vi "enable_disable.vi"(8 "error in (no error)":errorcluster, 9 "state":T3(ring), 10 "controls":T2[](array[typedef]), 11 "control references in":T1) -> (0 "error out":errorcluster, 3 "control references out":T1)   [LabVIEW 2010]
uses:
  type_definitions/enumerations/main_control_types.ctl
  type_definitions/clusters/controls_refs.ctl
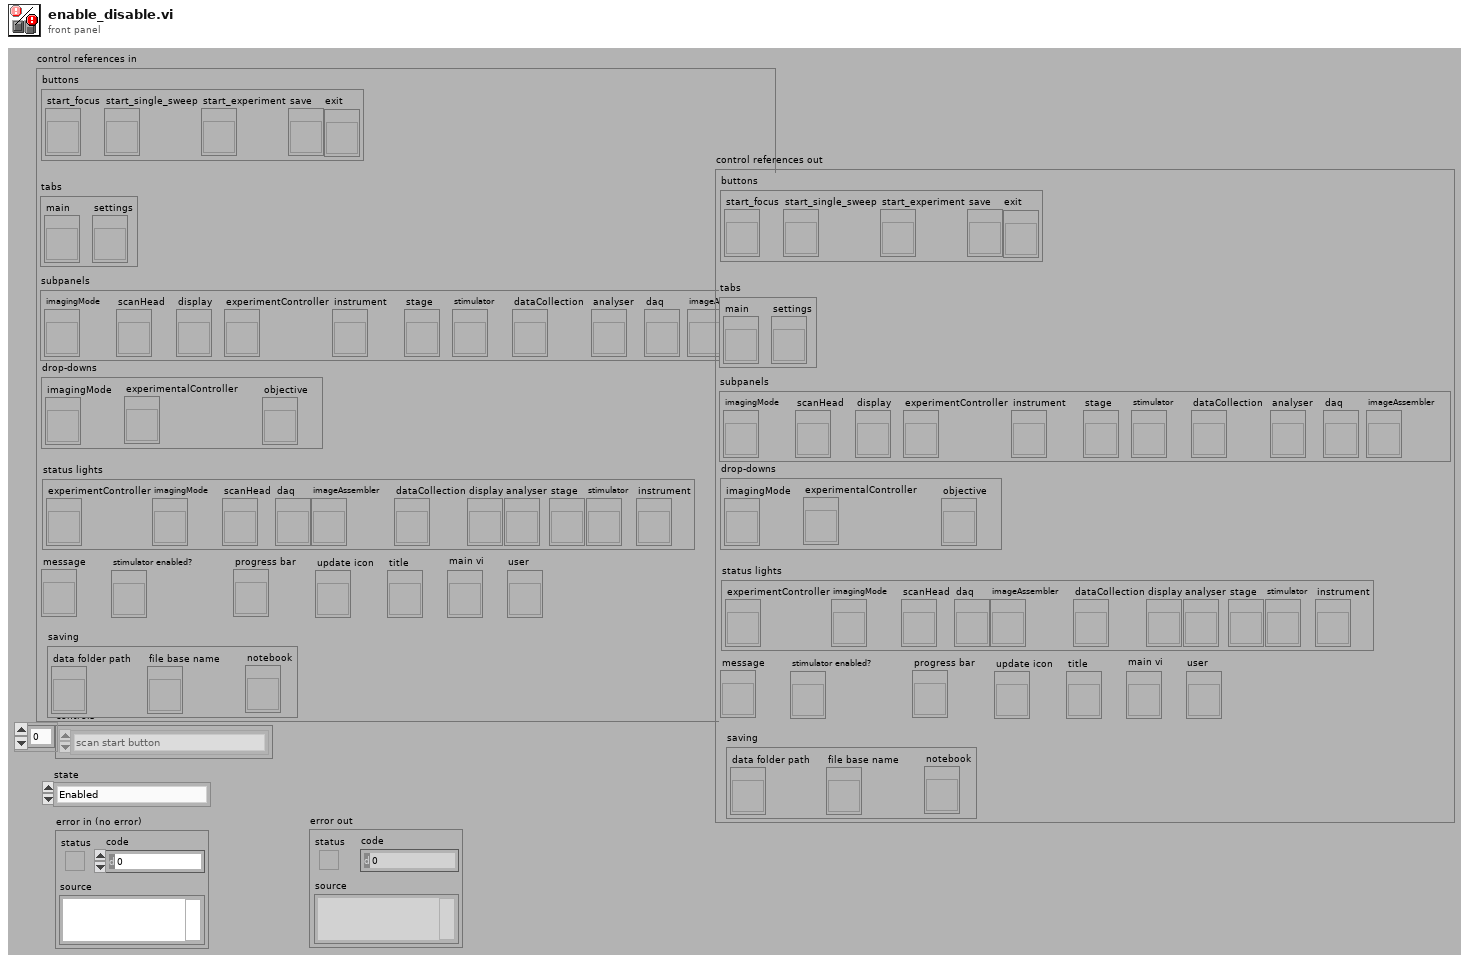
[diagram p1: front panel]
types:
  T1 = typedef "controls_refs.ctl" = cluster{"buttons":cluster{"start_focus":refnum<vi>, "start_single_sweep":refnum<vi>, "start_experiment":refnum<vi>, "save":refnum<vi>, "exit":refnum<vi>}, "tabs":cluster{"main":refnum<vi>, "settings":refnum<vi>}, "subpanels":cluster{"imagingMode":refnum<vi>, "scanHead":refnum<vi>, "display":refnum<vi>, "experimentController":refnum<vi>, "instrument":refnum<vi>, "stage":refnum<vi>, "stimulator":refnum<vi>, "dataCollection":refnum<vi>, "analyser":refnum<vi>, "daq":refnum<vi>, "imageAssembler":refnum<vi>}, "drop-downs":cluster{"imagingMode":refnum<vi>, "experimentalController":refnum<vi>, "objective":refnum<vi>}, "status lights":cluster{"experimentController":refnum<vi>, "imagingMode":refnum<vi>, "scanHead":refnum<vi>, "daq":refnum<vi>, "imageAssembler":refnum<vi>, "dataCollection":refnum<vi>, "display":refnum<vi>, "analyser":refnum<vi>, "stage":refnum<vi>, "stimulator":refnum<vi>, "instrument":refnum<vi>}, "message":refnum<vi>, "stimulator enabled?":refnum<vi>, "saving":cluster{"data folder path":refnum<vi>, "file base name":refnum<vi>, "notebook":refnum<vi>}, "progress bar":refnum<vi>, "update icon":refnum<vi>, "title":refnum<vi>, "main vi":refnum<vi>, "user":refnum<vi>}
  T2 = typedef "main_control_types.ctl" = enum16{"scan start button", "experimentController subpanel", "imagingMode subpanel", "scanHead subpanel", "dataCollection subpanel", "display subpanel", "analyser subpanel", "stimulator subpanel", "imagingMode drop-down", "experimentController drop-down", "objective drop-down", "exit button"}
  T3 = enum8{"Enabled", "Disabled", "Disabled and Grayed Out"}
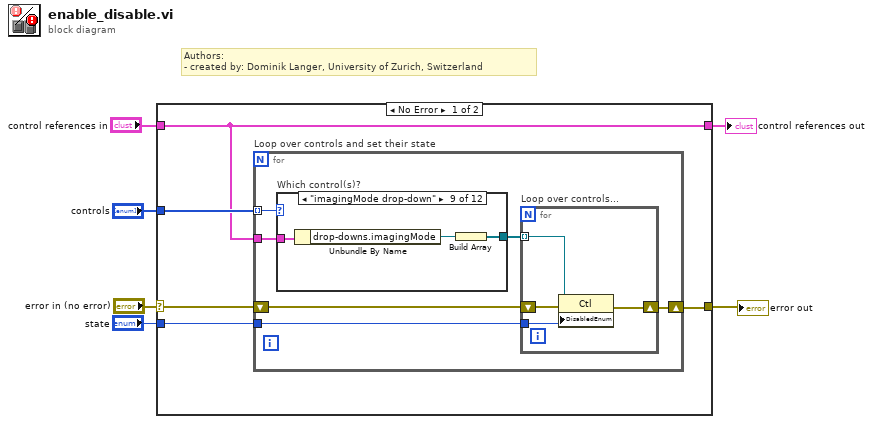
[diagram p0: block diagram]
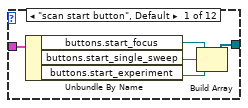
[diagram p2: hidden frame]
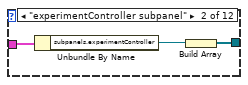
[diagram p3: hidden frame]
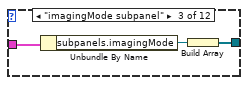
[diagram p4: hidden frame]
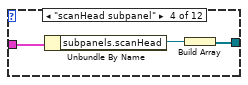
[diagram p5: hidden frame]
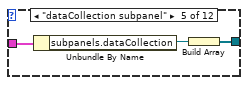
[diagram p6: hidden frame]
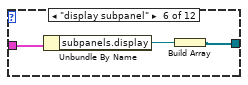
[diagram p7: hidden frame]
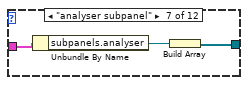
[diagram p8: hidden frame]
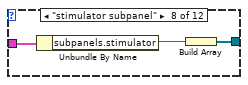
[diagram p9: hidden frame]
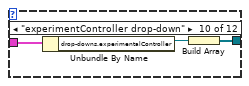
[diagram p10: hidden frame]
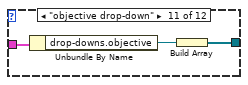
[diagram p11: hidden frame]
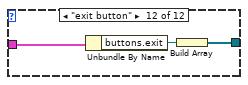
[diagram p12: hidden frame]
diagram:
  # "Authors: \n- created by: Dominik Langer, University of Zurich, Switzerland"
  n1 = case shown="No Error" "error in (no error)" {
    selector: "error in (no error)" -> [w8 w61]
    tunnel: [w10 w61] -> w5
    tunnel: "state" -> [w11 _]
    tunnel: "controls" -> [w9 _]
    tunnel: "control references in" -> [w7 w60]
    tunnel: [w7 w60] -> w1
    frame No Error {
      n2 = for "Loop over controls and set their state" {
        tunnel: w7 -> [w17]
        tunnel: w11 -> [w14]
        tunnel: w9 -> [w12] mode=indexing
        shift-right: [w13] -> w10
        shift-left: w8 -> [w16]
        n3 = case "Which control(s)?" shown="\"imagingMode drop-down\"" w12 {
          tunnel: w17 -> [w26 w29 w32 w35 w38 w41 w44 w47 w50 w53 w56 w59]
          tunnel: [w22 w27 w30 w34 w37 w39 w42 w45 w48 w52 w54 w57] -> w15
          frame "scan start button", Default {
            n4 = Unbundle By Name(w26) -> ("buttons.start_focus"=w24:refnum<vi>, "buttons.start_single_sweep"=w23:refnum<vi>, "buttons.start_experiment"=w25:refnum<vi>)
            n5 = Build Array(w24, w23, w25) -> (w22:refnum<vi>[])
          }
          frame "experimentController subpanel" {
            n6 = Unbundle By Name(w29) -> ("subpanels.experimentController"=w28:refnum<vi>)
            n7 = Build Array(w28) -> (w27:refnum<vi>[])
          }
          frame "imagingMode subpanel" {
            n8 = Unbundle By Name(w32) -> ("subpanels.imagingMode"=w31:refnum<vi>)
            n9 = Build Array(w31) -> (w30:refnum<vi>[])
          }
          frame "scanHead subpanel" {
            n10 = Unbundle By Name(w35) -> ("subpanels.scanHead"=w33:refnum<vi>)
            n11 = Build Array(w33) -> (w34:refnum<vi>[])
          }
          frame "dataCollection subpanel" {
            n12 = Unbundle By Name(w38) -> ("subpanels.dataCollection"=w36:refnum<vi>)
            n13 = Build Array(w36) -> (w37:refnum<vi>[])
          }
          frame "display subpanel" {
            n14 = Unbundle By Name(w41) -> ("subpanels.display"=w40:refnum<vi>)
            n15 = Build Array(w40) -> (w39:refnum<vi>[])
          }
          frame "analyser subpanel" {
            n16 = Unbundle By Name(w44) -> ("subpanels.analyser"=w43:refnum<vi>)
            n17 = Build Array(w43) -> (w42:refnum<vi>[])
          }
          frame "stimulator subpanel" {
            n18 = Unbundle By Name(w47) -> ("subpanels.stimulator"=w46:refnum<vi>)
            n19 = Build Array(w46) -> (w45:refnum<vi>[])
          }
          frame "imagingMode drop-down" {
            n20 = Unbundle By Name(w50) -> ("drop-downs.imagingMode"=w49:refnum<vi>)
            n21 = Build Array(w49) -> (w48:refnum<vi>[])
          }
          frame "experimentController drop-down" {
            n22 = Unbundle By Name(w53) -> ("drop-downs.experimentalController"=w51:refnum<vi>)
            n23 = Build Array(w51) -> (w52:refnum<vi>[])
          }
          frame "objective drop-down" {
            n24 = Unbundle By Name(w56) -> ("drop-downs.objective"=w55:refnum<vi>)
            n25 = Build Array(w55) -> (w54:refnum<vi>[])
          }
          frame "exit button" {
            n26 = Unbundle By Name(w59) -> ("buttons.exit"=w58:refnum<vi>)
            n27 = Build Array(w58) -> (w57:refnum<vi>[])
          }
        }
        n28 = for "Loop over controls..." {
          tunnel: w15 -> [w20] mode=indexing
          tunnel: w14 -> [w19]
          shift-right: [w18] -> w13
          shift-left: w16 -> [w21]
          n29 = property class="Ctl"(reference=w20, error in=w21, "DisabledEnum"=w19) -> (error out=w18:errorcluster)  [unwired: 1 out]
        }
      }
    }
    frame Error {
    }
  }
  "error out" <- w5
  "control references out" <- w1
